vi "UMLEditor UpdateNewMenu.vi"(0 "menu":refnum<k9>, 2 "GraphTypes":refnum<class "Graph.lvclass">[](array[class]), 5 "error in (no error)":errorcluster) -> (19 "error out":errorcluster)   [LabVIEW 2016]
doc: "Gets current diagram values"
uses:
  <resource>/Framework/Providers/Open_GDS/UML/Graph_class/Graph.lvclass
  <vilib>/Utility/miscctls.llb/LVMenuShortCut.ctl
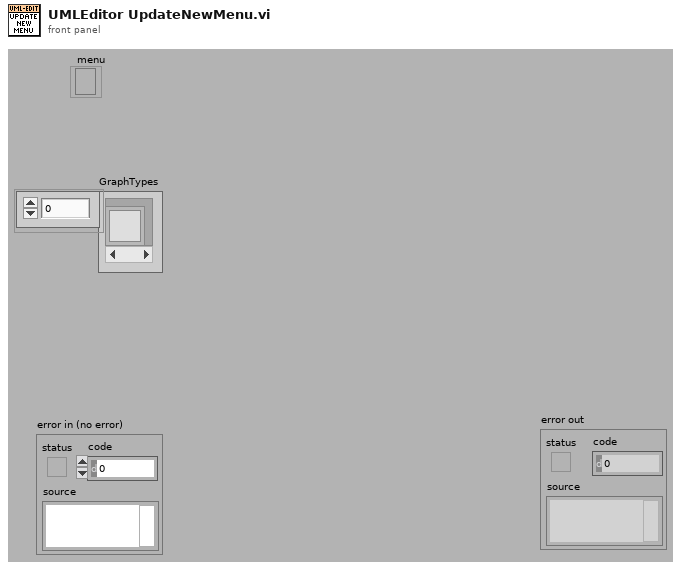
[diagram p1: front panel]
types:
  T1 = typedef "LVMenuShortCut.ctl" = cluster{"Include Shift Key?":bool, "Include Ctrl Key?":bool, "Shortcut Key":string}
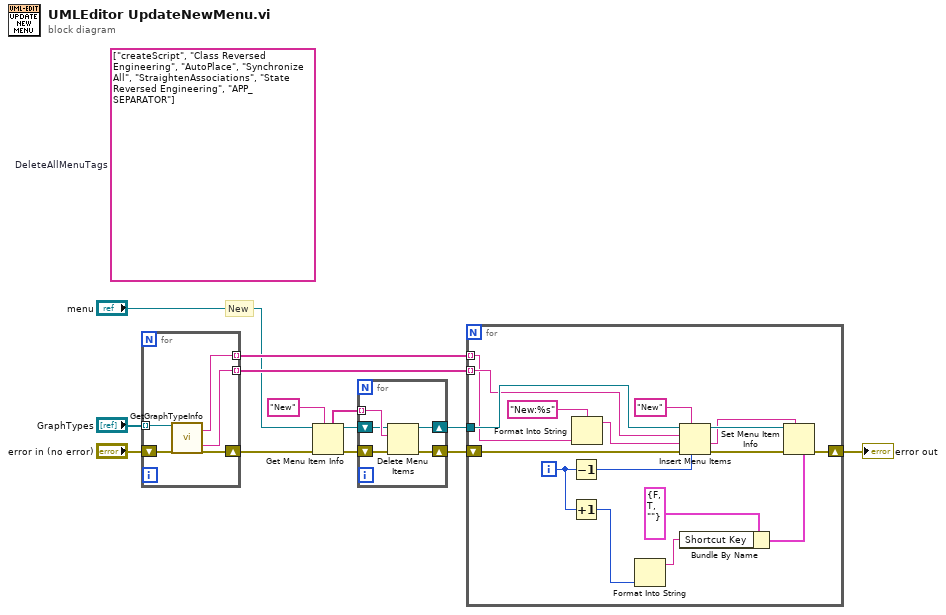
[diagram p0: block diagram]
diagram:
  (unwired) string[] ["createScript", "Class Reversed Engineering", "AutoPlace", "Synchronize All", "StraightenAssociations", "State Reversed Engineering", "APP_SEPARATOR"]  # DeleteAllMenuTags
  # "New"
  n1 = for {
    shift-right: [w17] -> w7
    shift-left: "error in (no error)" -> [w18]
    tunnel: "GraphTypes" -> [w16] mode=indexing
    tunnel: [w15] -> w11 mode=indexing
    tunnel: [w14] -> w10 mode=indexing
    n2 = call-dynamic "GetGraphTypeInfo.vi"("reference in"=w16, "error in (no error)"=w18) -> ("GraphTypeName"=w14:string, "GraphTypeUserName"=w15:string, "error out"=w17:errorcluster)  [unwired: 12 in, 3 out]
  }
  n3 = Get Menu Item Info(7:"New" ("item tag"), 8:w7, 11:"menu") -> (0:w4:errorcluster, 3:w5:refnum<k9>, 5:w6:string[])  [unwired: 4 out]
  n4 = for {
    tunnel: w6 -> [w23] mode=indexing
    shift-right: [w20] -> w2
    shift-left: w4 -> [w21]
    shift-right: [w19] -> w3
    shift-left: w5 -> [w22]
    n5 = Delete Menu Items(6:w21, 8:w23, 9:w22) -> (0:w20:errorcluster, 3:w19:refnum<k9>)  [unwired: 1 in]
  }
  n6 = for {
    shift-right: [w36] -> w1
    shift-left: w2 -> [w38]
    tunnel: w3 -> [w37]
    tunnel: w11 -> [w33] mode=indexing
    tunnel: w10 -> [w24] mode=indexing
    i -> [w26]
    n7 = Decrement(x=w26) -> (x-1=w34:i32)
    n8 = Increment(x=w26) -> (x+1=w29:i32)
    n9 = Format Into String(format string="New:%s" ("menu tag"), w24) -> (resulting string=w25:string)  [unwired: 2 in, 1 out]
    n10 = Format Into String(w29) -> (resulting string=w28:string)  [unwired: 3 in, 1 out]
    n11 = Insert Menu Items(4:w34, 5:"New" ("menu tag"), 6:w38, 7:w25, 8:w33, 9:w37) -> (0:w35:errorcluster, 1:w32:string, 3:w39:refnum<k9>)
    n12 = Bundle By Name(cluster=T1 {"Include Shift Key?"=FALSE, "Include Ctrl Key?"=TRUE, "Shortcut Key"=""} ("short cut"), "Shortcut Key"=w28) -> (w30:T1)
    n13 = Set Menu Item Info(4:w30, 7:w32, 8:w35, 11:w39) -> (0:w36:errorcluster)  [unwired: 4 out]
  }
  "error out" <- w1
